vi "getVP.vi"(7 "Reading type":T1, 8 "error in (no error)":errorcluster, 11 "VISA resource name":refnum<visa-resource-name>) -> (0 "error out":errorcluster, 1 "Pressure, Torr":dbl, 2 "Voltage, mV":dbl, 3 "VISA resource name out":refnum<visa-resource-name>)   [LabVIEW 2012, in "ValveController.lvlib"]
doc: "Runs the instrument's self-test routine and returns the test results."
uses:
  <instrlib>/ValveController/Public/Utility/EnumVoltPressType.ctl
  <instrlib>/ValveController/ValveController.lvlib
panel:
  out "read buffer":string
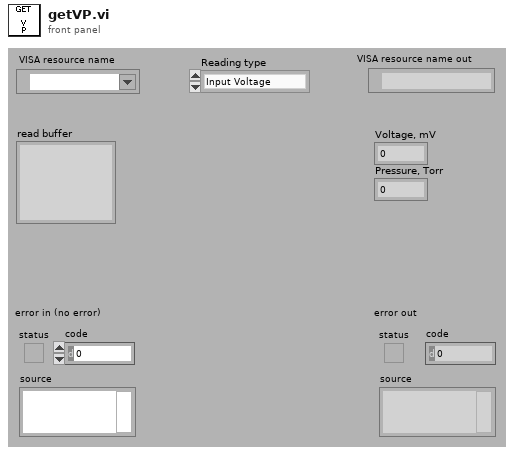
[diagram p1: front panel]
types:
  T1 = typedef "EnumVoltPressType.ctl" = enum16{"Input Voltage", "Hw threshold voltage", "Sw threshold voltage"}
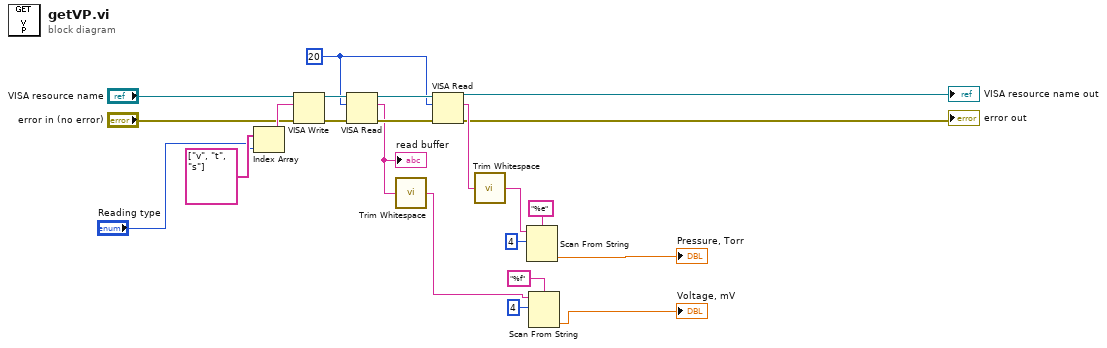
[diagram p0: block diagram]
diagram:
  w18 = u32 20 ("byte count (20)")
  n1 = Index Array(array=string[] ["v", "t", "s"], index="Reading type") -> (element=w8:string)
  n2 = VISA Write(VISA resource name="VISA resource name", write buffer=w8, error in (no error)="error in (no error)") -> (VISA resource name out=w22:refnum<visa-resource-name>, error out=w21:errorcluster)  [unwired: 1 out]
  n3 = VISA Read(VISA resource name=w22, byte count=w18, error in (no error)=w21) -> (VISA resource name out=w19:refnum<visa-resource-name>, read buffer=w13:string, error out=w20:errorcluster)  [unwired: 1 out]
  "read buffer" <- w13
  n4 = call <vilib>:"Trim Whitespace.vi"("string"=w13) -> ("trimmed string"=w12:string)  [unwired: 1 in]
  n5 = VISA Read(VISA resource name=w19, byte count=w18, error in (no error)=w20) -> (VISA resource name out=→"VISA resource name out":refnum<visa-resource-name>, read buffer=w11:string, error out=→"error out":errorcluster)  [unwired: 1 out]
  n6 = call <vilib>:"Trim Whitespace.vi"("string"=w11) -> ("trimmed string"=w10:string)  [unwired: 1 in]
  n7 = Scan From String(format string="%e", input string=w10, initial scan location=u32 4) -> (output 1=→"Pressure, Torr":dbl)  [unwired: 2 in, 3 out]
  n8 = Scan From String(format string="%f", input string=w12, initial scan location=u32 4) -> (output 1=→"Voltage, mV":dbl)  [unwired: 2 in, 3 out]
